vi "TimeInterpBoolean_Clear.vi"(11 "in TimeInterpBoolean":T1) -> (3 "out TimeInterpBoolean":T1)   [LabVIEW 2019, in "Trajectory_Library.lvlib"]
doc: "Removes all samples from the history buffer.\n\nInputs:\n - In TimeInterpBoolean -- Input data cluster.\n\nOutputs:\n - Out TimeInterpBoolean -- Updated data cluster."
uses:
  Trajectory_Library.lvlib
  TIME_INTERPOLATABLE_BOOLEAN.ctl
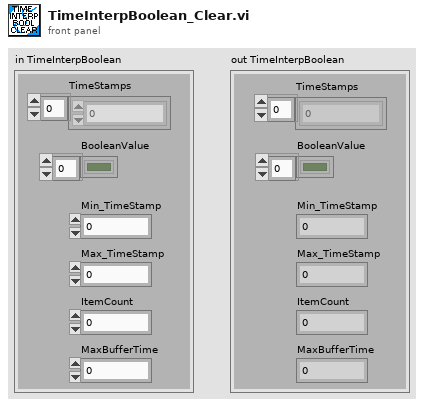
[diagram p1: front panel]
types:
  T1 = typedef "Trajectory_Library.lvlib/TIME_INTERPOLATABLE_BOOLEAN.ctl" = cluster{"TimeStamps":dbl[], "BooleanValue":bool[], "Min_TimeStamp":dbl, "Max_TimeStamp":dbl, "ItemCount":i32, "MaxBufferTime":dbl}
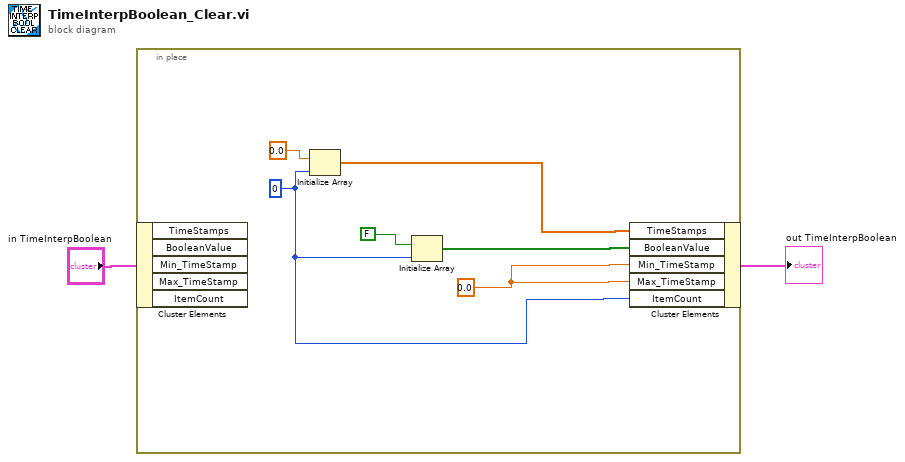
[diagram p0: block diagram]
diagram:
  n1 = in-place {
    w5 = 0.0 ("X")
    w4 = 0 ("dimension size")
    n2 = in-place-cluster #1("in TimeInterpBoolean") -> ()  [unwired: 5 out]
    n3 = Initialize Array(0.0 ("element"), w4) -> (w7:dbl[])
    n4 = Initialize Array(FALSE, w4) -> (w6:bool[])
    n5 = in-place-cluster #1("TimeStamps"=w7, "BooleanValue"=w6, "Min_TimeStamp"=w5, "Max_TimeStamp"=w5, "ItemCount"=w4) -> (→"out TimeInterpBoolean":T1)
  }
